vi "Facade.vi"(0 "Data In":T4={"Active"=FALSE, "Delay (ms)"=0.0, "Duration (ms)"=50.0, "Ramp (ms)"=5.0, "Rate (Hz)"=0.0, "Trepeat (ms)"=0.0, "Repeat"=FALSE}, 2 "Display State In":T2, 3 "Container State":T3) -> (6 "Data Out":T4={"Active"=FALSE, "Delay (ms)"=0.0, "Duration (ms)"=50.0, "Ramp (ms)"=5.0, "Rate (Hz)"=0.0, "Trepeat (ms)"=0.0, "Repeat"=FALSE}, 7 "Display State Out":T2, 8 "Action":T1)   [LabVIEW 2020, in "Burst (G3).xctl"]
uses:
  Burst (G3).xctl
  Burst Data.ctl
  <vilib>/_xctls/Container State.ctl
  State.ctl
  Utility VIs/Controls/KCheckbox/KCheckbox.xctl
  Utility VIs/Controls/KNumeric (DBL)/KNumeric (DBL).xctl
  <vilib>/_xctls/Action.ctl
  <vilib>/_xctls/XControlSupport.lvlib
panel:
  out "redisplay":bool
  in  "Ramp (ms)":dbl(xcontrol)
  in  "Duration (ms)":dbl(xcontrol)
  in  "Active":bool(xcontrol) caption="Gated?"
  in  "Delay (ms)":dbl(xcontrol)
  in  "for":dbl(xcontrol) caption="ms"
  in  "at":dbl(xcontrol) caption="Hz"
  in  "Repeat":bool(xcontrol)
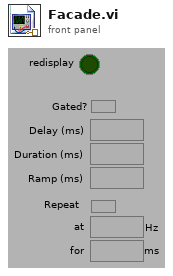
[diagram p1: front panel]
types:
  T1 = typedef "XControlSupport.lvlib/Action.ctl" = cluster{"Data Changed?":bool, "State Changed?":bool, "Action Name":string}
  T2 = typedef "Burst (G3).xctl/State.ctl" = cluster{"ctls":cluster{"Active":refnum<vi>, "Delay":refnum<vi>, "Dur":refnum<vi>, "Ramp":refnum<vi>, "Repeat":refnum<vi>, "at":refnum<vi>, "for":refnum<vi>}, "active mixed":bool, "repeat mixed":bool}
  T3 = typedef "XControlSupport.lvlib/Container State.ctl" = cluster{"Indicator?":bool, "Run Mode?":bool, " Refnum":refnum<vi>}
  T4 = typedef "Burst (G3).xctl/Burst Data.ctl" = cluster{"Active":bool, "Delay (ms)":dbl, "Duration (ms)":dbl, "Ramp (ms)":dbl, "Rate (Hz)":dbl, "Trepeat (ms)":dbl, "Repeat":bool}
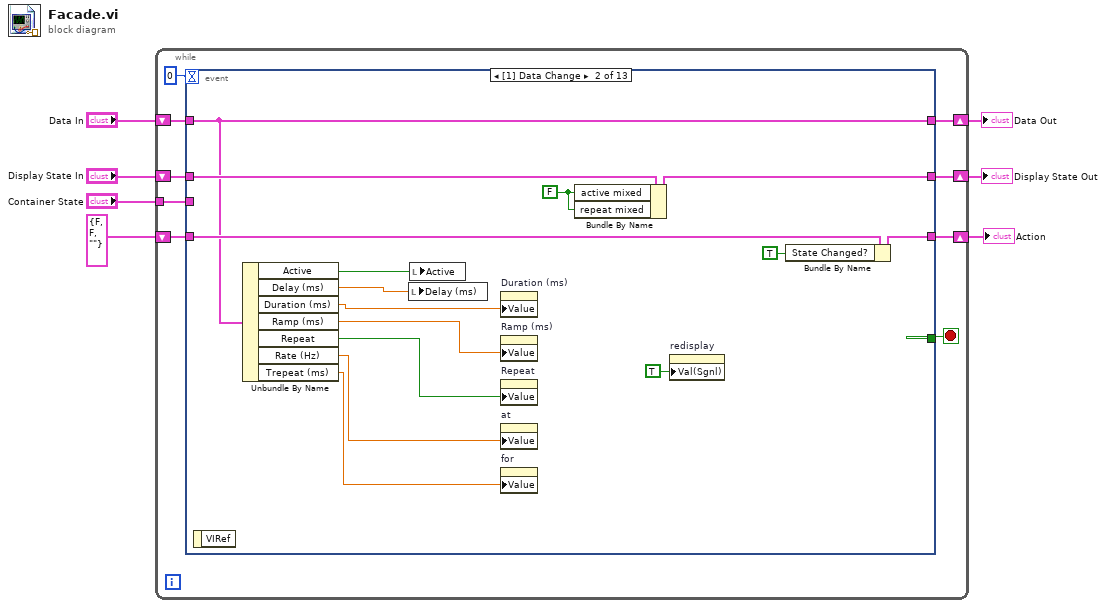
[diagram p0: block diagram]
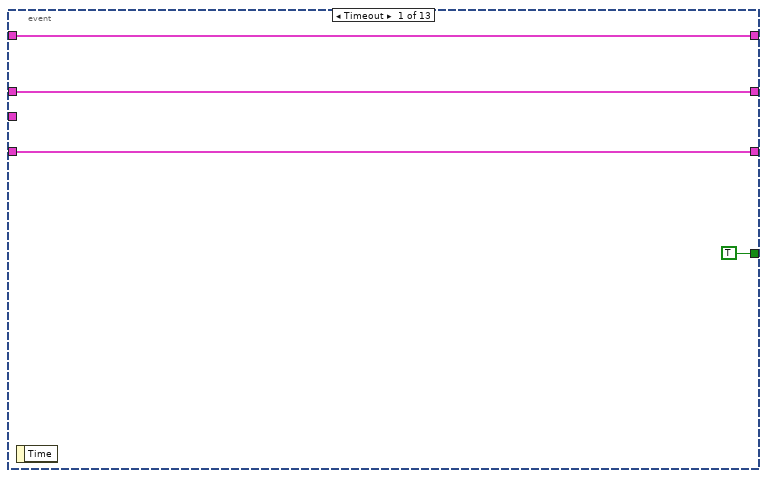
[diagram p2: hidden frame]
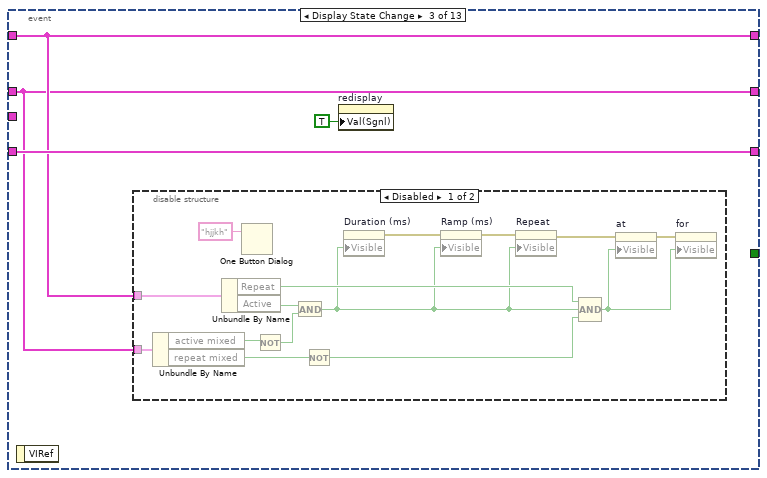
[diagram p3: hidden frame]
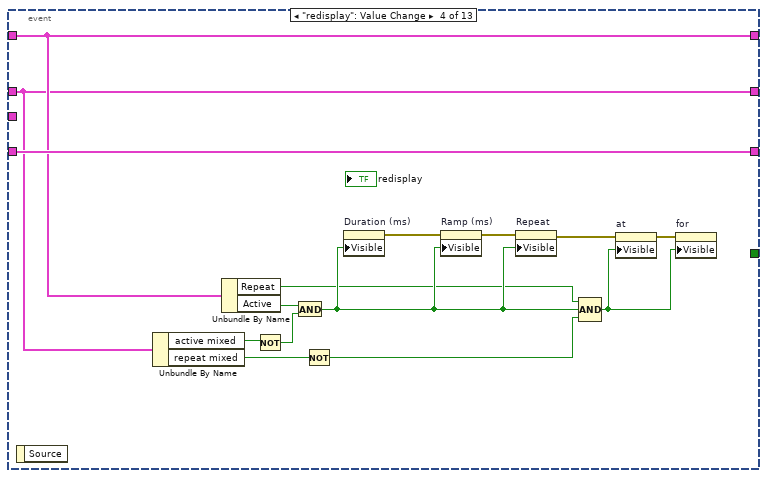
[diagram p5: hidden frame]
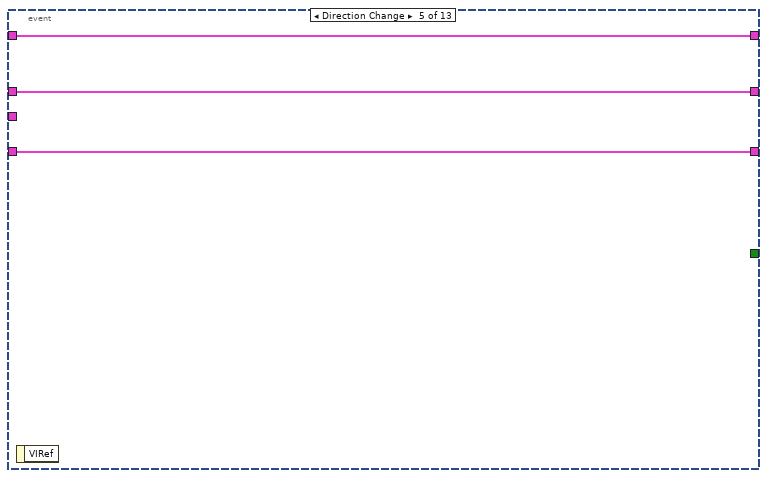
[diagram p6: hidden frame]
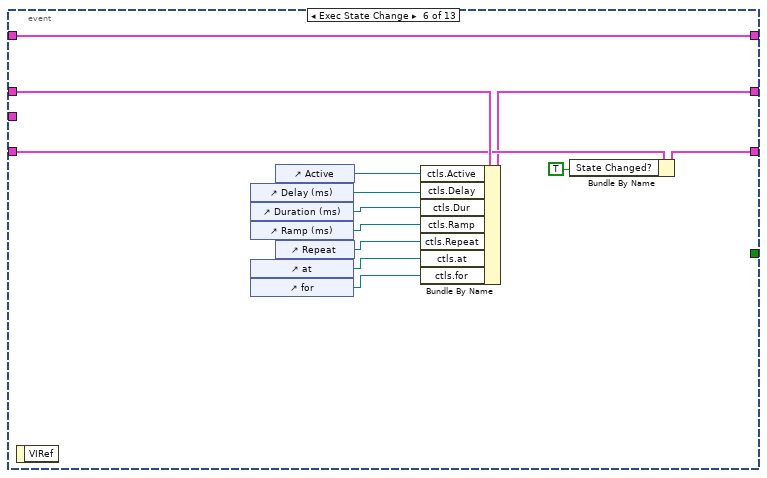
[diagram p7: hidden frame]
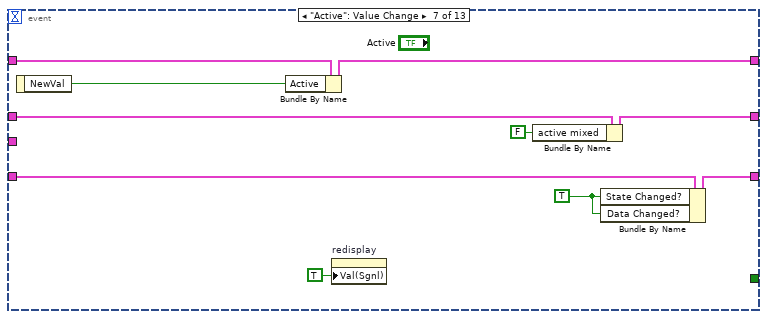
[diagram p8: hidden frame]
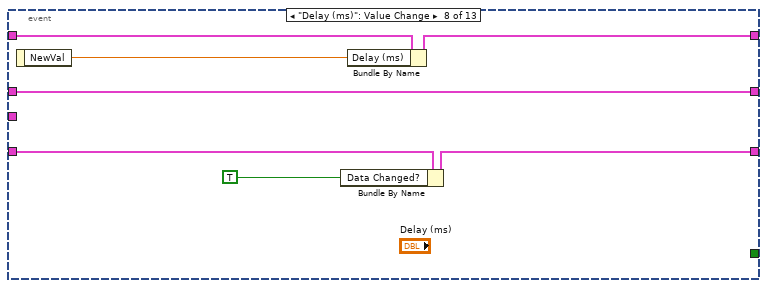
[diagram p9: hidden frame]
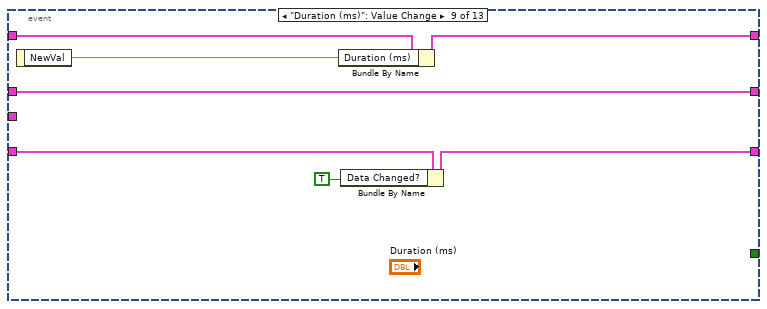
[diagram p10: hidden frame]
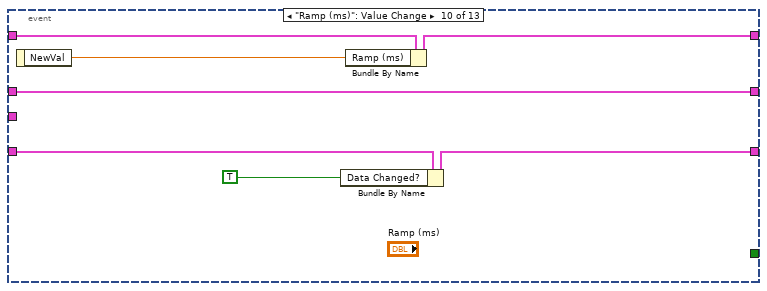
[diagram p11: hidden frame]
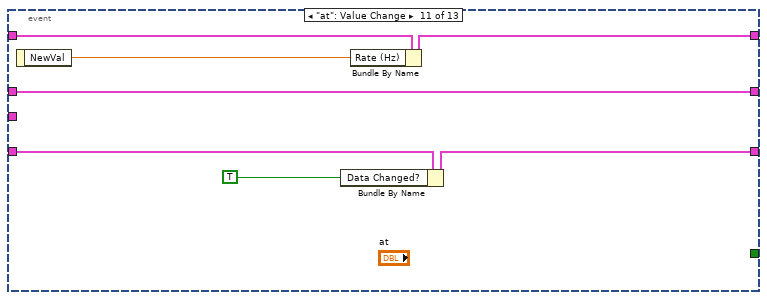
[diagram p12: hidden frame]
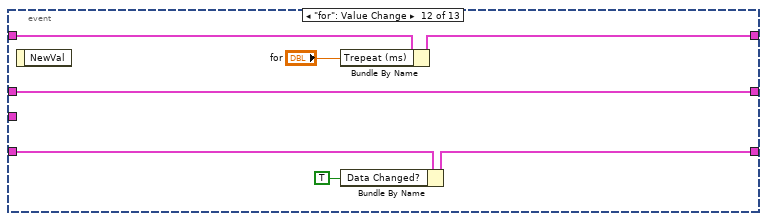
[diagram p13: hidden frame]
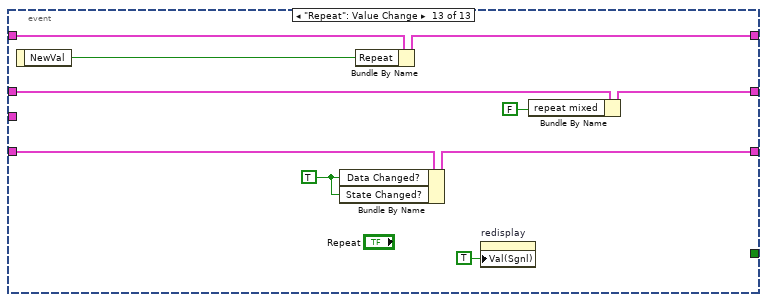
[diagram p14: hidden frame]
diagram:
  n1 = while {
    shift-right: [w15] -> w4
    shift-left: "Display State In" -> [w16]
    tunnel: "Container State" -> [w12]
    shift-right: [w10] -> w7
    shift-left: "Data In" -> [w11]
    shift-right: [w8] -> w2
    shift-left: T1 {"Data Changed?"=FALSE, "State Changed?"=FALSE, "Action Name"=""} ("Action") -> [w9]
    stop <- w14 stop-if-true
    n2 = event shown="[1] Data Change" {
      selector: _ -> [_ _ _ _ _ _ _ _ _ _ _ _ _]
      dyn-events: _ -> [_ _ _ _ _ _ _ _ _ _ _ _ _]
      timeout: 0 -> [_ _ _ _ _ _ _ _ _ _ _ _ _]
      tunnel: w16 -> [w18 w35 w37 w67 w72 w85 w90 w102 w109 w116 w123 w130 w140]
      tunnel: [w18 w32 w37 w67 w72 w82 w89 w102 w109 w116 w123 w130 w134] -> w15
      tunnel: [TRUE _ _ _ _ _ _ _ _ _ _ _ _] -> w14
      tunnel: w12 -> [_ _ _ _ _ _ _ _ _ _ _ _ _]
      tunnel: w11 -> [w17 w33 w38 w68 w71 w84 w92 w98 w105 w112 w119 w126 w137]
      tunnel: [w17 w33 w38 w68 w71 w84 w93 w96 w103 w110 w117 w125 w135] -> w10
      tunnel: [w19 w30 w39 w69 w70 w74 w94 w100 w107 w114 w121 w128 w138] -> w8
      tunnel: w9 -> [w19 w34 w39 w69 w70 w83 w95 w101 w108 w115 w122 w129 w139]
      event Timeout {
        n3 = event-data() -> ()  [unwired: 1 in, 1 out]
      }
      event Data Change {
        w31 = FALSE ("active mixed")
        n4 = event-data() -> ()  [unwired: 1 in, 1 out]
        n5 = Unbundle By Name(w33) -> ("Active"=w28:bool, "Delay (ms)"=w27:dbl, "Duration (ms)"=w26:dbl, "Ramp (ms)"=w24:dbl, "Repeat"=w22:bool, "Rate (Hz)"=w23:dbl, "Trepeat (ms)"=w21:dbl)
        n6 = local write "Delay (ms)"(w27) -> ()
        n7 = local write "Active"(w28) -> ()
        n8 = property on="Duration (ms)" class="KNumeric (DBL) (strict)"("Value"=w26) -> ()  [unwired: 2 in, 2 out]
        n9 = property on="Ramp (ms)" class="KNumeric (DBL) (strict)"("Value"=w24) -> ()  [unwired: 2 in, 2 out]
        n10 = property on="Repeat" class="KCheckbox (strict)"("Value"=w22) -> ()  [unwired: 2 in, 2 out]
        n11 = property on="at" class="KNumeric (DBL) (strict)"("Value"=w23) -> ()  [unwired: 2 in, 2 out]
        n12 = property on="for" class="KNumeric (DBL) (strict)"("Value"=w21) -> ()  [unwired: 2 in, 2 out]
        n13 = Bundle By Name(cluster=w35, "active mixed"=w31, "repeat mixed"=w31) -> (w32:T2)
        n14 = property on="redisplay" class="Bool (strict)"("Val(Sgnl)"=TRUE ("Value (Signaling)")) -> ()  [unwired: 2 in, 2 out]
        n15 = Bundle By Name(cluster=w34, "State Changed?"=TRUE) -> (w30:T1)
      }
      event Display State Change {
        n16 = event-data() -> ()  [unwired: 1 in, 1 out]
        n17 = disable-structure shown="Disabled" {
          disable-tunnel: w38 -> [w54 _]
          disable-tunnel: w37 -> [w53 _]
          frame Disabled {
            n18 = Unbundle By Name(w53) -> ("active mixed"=w47:bool, "repeat mixed"=w46:bool)
            n19 = Unbundle By Name(w54) -> ("Repeat"=w43:bool, "Active"=w45:bool)
            n20 = One Button Dialog(message="hjjkh") -> ()  [unwired: 1 in, 1 out]
            n21 = Not(x=w47) -> (.not. x?=w44:bool)
            n22 = And(x=w45, y=w44) -> (x .and. y?=w41:bool)
            n23 = Not(x=w46) -> (.not. x?=w42:bool)
            n24 = property on="Duration (ms)" class="KNumeric (DBL) (strict)"("Visible"=w41) -> (error out=w52:errorcluster)  [unwired: 2 in, 1 out]
            n25 = property on="Ramp (ms)" class="KNumeric (DBL) (strict)"(error in=w52, "Visible"=w41) -> (error out=w51:errorcluster)  [unwired: 1 in, 1 out]
            n26 = property on="Repeat" class="KCheckbox (strict)"(error in=w51, "Visible"=w41) -> (error out=w50:errorcluster)  [unwired: 1 in, 1 out]
            n27 = Compound Arithmetic op=AND(w43, w41, w42) -> (w48:bool)
            n28 = property on="at" class="KNumeric (DBL) (strict)"(error in=w50, "Visible"=w48) -> (error out=w49:errorcluster)  [unwired: 1 in, 1 out]
            n29 = property on="for" class="KNumeric (DBL) (strict)"(error in=w49, "Visible"=w48) -> ()  [unwired: 1 in, 2 out]
          }
          frame Enabled {
          }
        }
        n30 = property on="redisplay" class="Bool (strict)"("Val(Sgnl)"=TRUE ("Value (Signaling)")) -> ()  [unwired: 2 in, 2 out]
      }
      event "redisplay": Value Change {
        n31 = event-data() -> ()  [unwired: 1 in, 1 out]
        n32 = Unbundle By Name(w67) -> ("active mixed"=w61:bool, "repeat mixed"=w60:bool)
        n33 = Unbundle By Name(w68) -> ("Repeat"=w55:bool, "Active"=w59:bool)
        n34 = Not(x=w61) -> (.not. x?=w58:bool)
        n35 = And(x=w59, y=w58) -> (x .and. y?=w56:bool)
        n36 = Not(x=w60) -> (.not. x?=w57:bool)
        n37 = property on="Duration (ms)" class="KNumeric (DBL) (strict)"("Visible"=w56) -> (error out=w66:errorcluster)  [unwired: 2 in, 1 out]
        n38 = property on="Ramp (ms)" class="KNumeric (DBL) (strict)"(error in=w66, "Visible"=w56) -> (error out=w65:errorcluster)  [unwired: 1 in, 1 out]
        n39 = property on="Repeat" class="KCheckbox (strict)"(error in=w65, "Visible"=w56) -> (error out=w64:errorcluster)  [unwired: 1 in, 1 out]
        n40 = Compound Arithmetic op=AND(w55, w56, w57) -> (w62:bool)
        n41 = property on="at" class="KNumeric (DBL) (strict)"(error in=w64, "Visible"=w62) -> (error out=w63:errorcluster)  [unwired: 1 in, 1 out]
        n42 = property on="for" class="KNumeric (DBL) (strict)"(error in=w63, "Visible"=w62) -> ()  [unwired: 1 in, 2 out]
      }
      event Direction Change {
        n43 = event-data() -> ()  [unwired: 1 in, 1 out]
      }
      event Exec State Change {
        n44 = event-data() -> ()  [unwired: 1 in, 1 out]
        n45 = control-ref of="Delay (ms)"() -> (w80:refnum<vi>)
        n46 = control-ref of="Duration (ms)"() -> (w79:refnum<vi>)
        n47 = control-ref of="Ramp (ms)"() -> (w78:refnum<vi>)
        n48 = control-ref of="at"() -> (w76:refnum<vi>)
        n49 = control-ref of="for"() -> (w75:refnum<vi>)
        n50 = control-ref of="Active"() -> (w81:refnum<vi>)
        n51 = control-ref of="Repeat"() -> (w77:refnum<vi>)
        n52 = Bundle By Name(cluster=w85, "ctls.Active"=w81, "ctls.Delay"=w80, "ctls.Dur"=w79, "ctls.Ramp"=w78, "ctls.Repeat"=w77, "ctls.at"=w76, "ctls.for"=w75) -> (w82:T2)
        n53 = Bundle By Name(cluster=w83, "State Changed?"=TRUE) -> (w74:T1)
      }
      event "Active": Value Change {
        w91 = TRUE ("State Changed?")
        n54 = event-data() -> ("NewVal"=w87:bool)  [unwired: 1 in]
        n55 = Bundle By Name(cluster=w92, "Active"=w87) -> (w93:T4)
        n56 = property on="redisplay" class="Bool (strict)"("Val(Sgnl)"=TRUE ("Value (Signaling)")) -> ()  [unwired: 2 in, 2 out]
        n57 = Bundle By Name(cluster=w90, "active mixed"=FALSE) -> (w89:T2)
        n58 = Bundle By Name(cluster=w95, "State Changed?"=w91, "Data Changed?"=w91) -> (w94:T1)
      }
      event "Delay (ms)": Value Change {
        n59 = event-data() -> ("NewVal"=w97:dbl)  [unwired: 1 in]
        n60 = Bundle By Name(cluster=w101, "Data Changed?"=TRUE) -> (w100:T1)
        n61 = Bundle By Name(cluster=w98, "Delay (ms)"=w97) -> (w96:T4)
      }
      event "Duration (ms)": Value Change {
        n62 = event-data() -> ("NewVal"=w104:dbl)  [unwired: 1 in]
        n63 = Bundle By Name(cluster=w105, "Duration (ms)"=w104) -> (w103:T4)
        n64 = Bundle By Name(cluster=w108, "Data Changed?"=TRUE) -> (w107:T1)
      }
      event "Ramp (ms)": Value Change {
        n65 = event-data() -> ("NewVal"=w111:dbl)  [unwired: 1 in]
        n66 = Bundle By Name(cluster=w115, "Data Changed?"=TRUE) -> (w114:T1)
        n67 = Bundle By Name(cluster=w112, "Ramp (ms)"=w111) -> (w110:T4)
      }
      event "at": Value Change {
        n68 = event-data() -> ("NewVal"=w118:dbl)  [unwired: 1 in]
        n69 = Bundle By Name(cluster=w122, "Data Changed?"=TRUE) -> (w121:T1)
        n70 = Bundle By Name(cluster=w119, "Rate (Hz)"=w118) -> (w117:T4)
      }
      event "for": Value Change {
        n71 = event-data() -> ()  [unwired: 1 in, 1 out]
        n72 = Bundle By Name(cluster=w126, "Trepeat (ms)"="for") -> (w125:T4)
        n73 = Bundle By Name(cluster=w129, "Data Changed?"=TRUE) -> (w128:T1)
      }
      event "Repeat": Value Change {
        w132 = TRUE ("Data Changed?")
        n74 = event-data() -> ("NewVal"=w136:bool)  [unwired: 1 in]
        n75 = Bundle By Name(cluster=w139, "Data Changed?"=w132, "State Changed?"=w132) -> (w138:T1)
        n76 = Bundle By Name(cluster=w137, "Repeat"=w136) -> (w135:T4)
        n77 = property on="redisplay" class="Bool (strict)"("Val(Sgnl)"=TRUE ("Value (Signaling)")) -> ()  [unwired: 2 in, 2 out]
        n78 = Bundle By Name(cluster=w140, "repeat mixed"=FALSE) -> (w134:T2)
      }
    }
  }
  "Display State Out" <- w4
  "Data Out" <- w7
  "Action" <- w2
